vi "save.vi"(7 "save raw data?":bool, 8 "error":errorcluster, 9 "calibration data":dbl[][](array[numeric]), 10 "measurement data":dbl[][](array[numeric]), 11 "tdms file":refnum<k34>) -> (0 "error out":errorcluster, 3 "tdms file out":refnum<k34>)   [LabVIEW 2017, in "Licor-Steuerung.lvlib"]
uses:
  Licor-Steuerung.lvlib
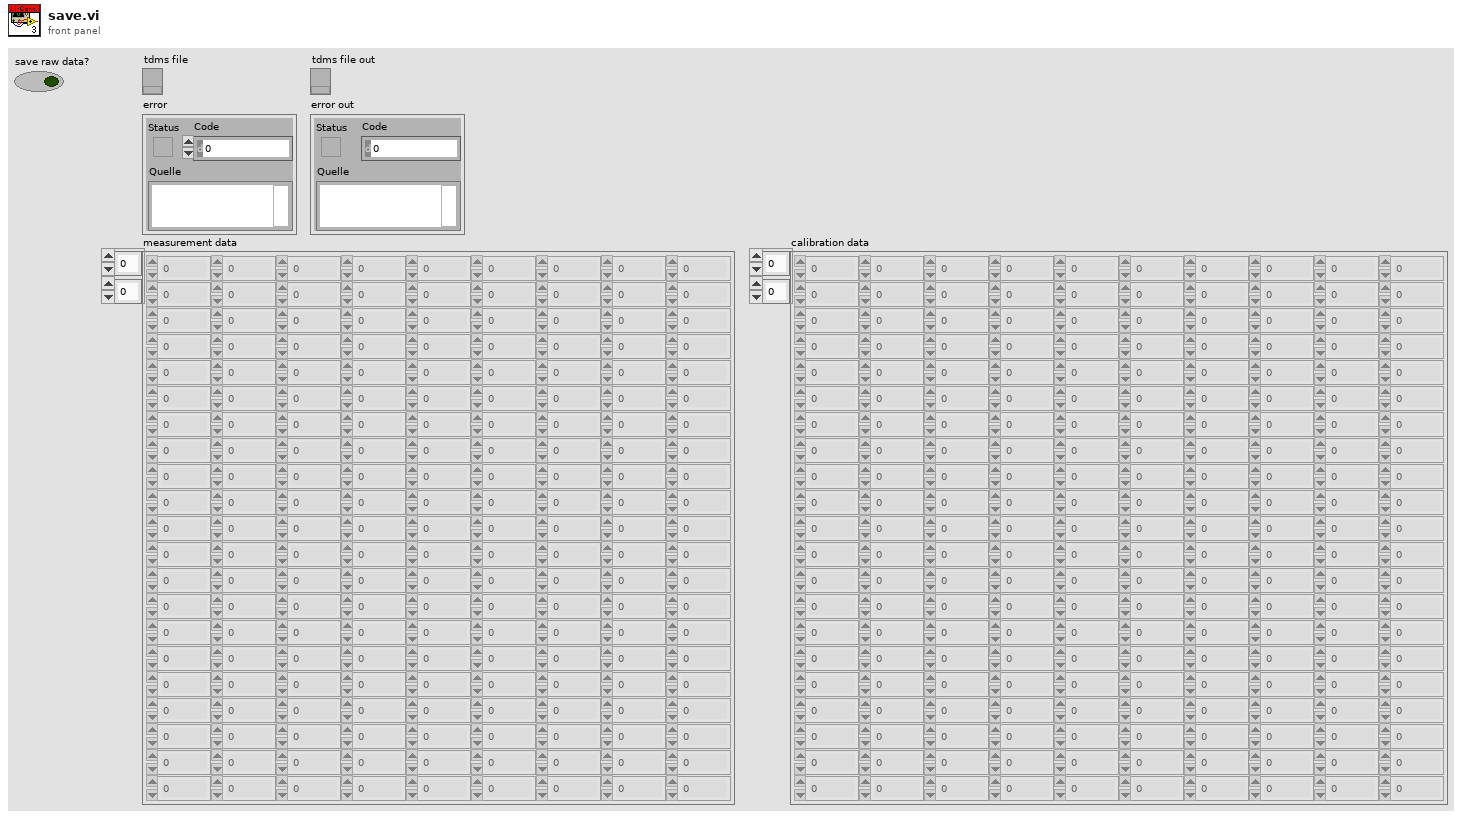
[diagram p1: front panel]
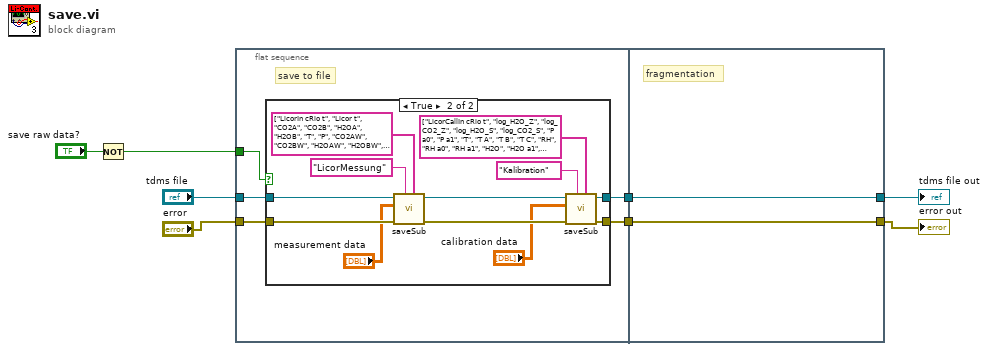
[diagram p0: block diagram]
diagram:
  n1 = Not(x="save raw data?") -> (.not. x?=w1:bool)
  n2 = flat-sequence {
    tunnel: "tdms file" -> [w13]
    tunnel: "error" -> [w12]
    tunnel: [w11] -> w6
    tunnel: [w10] -> w5
    tunnel: w1 -> [w9]
    tunnel: w6 -> [w29]
    tunnel: w5 -> [w28]
    tunnel: [w29] -> w4
    tunnel: [w28] -> w3
    frame #0 {
      # "save to file"
      n3 = case shown="True" w9 {
        tunnel: w13 -> [w15 w27]
        tunnel: w12 -> [w14 w26]
        tunnel: [w15 w17] -> w11
        tunnel: [w14 w16] -> w10
        frame False {
        }
        frame True {
          n4 = call "saveSub.vi"("Kanalnamen"=string[] ["LicorIn cRio t", "Licor t", "CO2A", "CO2B", "H2OA", "H2OB", "T", "P", "CO2AW", "CO2BW", "H2OAW", "H2OBW", "RH"] ("Kanalnamen (Eingang, unbenannt)"), "Gruppenname"="LicorMessung" ("Gruppenname (Eingang, Unbenannt)"), "error"=w26, "new data"="measurement data", "tdms file"=w27) -> ("error out"=w22:errorcluster, "tdms file out"=w23:refnum<k34>)  [unwired: 5 in]
          n5 = call "saveSub.vi"("Kanalnamen"=string[] ["LicorCallIn cRio t", "log_H2O_Z", "log_CO2_Z", "log_H2O_S", "log_CO2_S", "P a0", "P a1", "T", "T A", "T B", "T C", "RH", "RH a0", "RH a1", "H2O", "H2O a1", "H2O a2", "H2O a3", "H2O gamma", "H2O Z", "H2O Zt", "H2O Zm", "H2O S", "H2O W0", "H2O W0d", "H2O AGC", "CO2", "CO2 a1", "CO2 a2", "CO2 a3", "CO2 a4", "CO2 a5", "CO2 gamma", "CO2 Z", "CO2 Zt", "CO2 Zm", "CO2 S", "CO2 W0", "CO2 W0d", "CO2 AGC", "CO2 VpCrr"] ("Kanalnamen (Eingang, unbenannt)"), "Gruppenname"="Kalibration" ("Gruppenname (Eingang, Unbenannt)"), "error"=w22, "new data"="calibration data", "tdms file"=w23) -> ("error out"=w16:errorcluster, "tdms file out"=w17:refnum<k34>)  [unwired: 5 in]
        }
      }
    }
    frame #1 {
      # "fragmentation"
    }
  }
  "tdms file out" <- w4
  "error out" <- w3
